vi "Instrument Main Engine.vi"(10 "Parameters":variant, 11 "Process":refnum<class "Process.lvclass">) -> ()   [LabVIEW 2018, in "Instrument Addon Engine.lvlib"]
uses:
  Instrument Addon Engine.lvlib
  Addon Shared/Types/Linked Channel Cluster.ctl
  Addon Shared/Instrument Addon Shared.lvlib
  Addon Shared/Types/Command Parameters.ctl
  <vilib>/NI VeriStand/Custom Device API/Data Reference.ctl
  <vilib>/NI VeriStand/Custom Device API/Custom Device API.lvlib
  Addon Shared/Types/Response Wait Type.ctl
  Addon Shared/Types/Response Parameters.ctl
  Addon Shared/Types/Response RT Configuration Cluster.ctl
  Addon Shared/Types/Message Generation Type.ctl
  Addon Shared/Types/Message Parameters.ctl
  Addon Shared/Types/External Trigger Refs.ctl
  Addon Shared/Types/Compiled Settings.ctl
  niveristand-instrument-addon-custom-device/Source/Addon/Support Libraries/Protections.lvlibp/Parent Protection/Protection.lvclass
  niveristand-instrument-addon-custom-device/Source/Addon/Support Libraries/Protocols.lvlibp/Protocol Parent/Protocol Parent.lvclass
  Types/Commands RT Configuration Cluster.ctl
  <vilib>/NI/NI VeriStand Addon Network Comm/Engine/VeriStand Comm.lvclass
  Addon Shared/Types/Command Channel Index.ctl
  Addon Shared/Types/Command Channel Indeces.ctl
  <vilib>/NI/NIVS Inline Async API/_VS Inline Async API/Process/Process.lvclass
panel:
  in  "error in (no error)":errorcluster
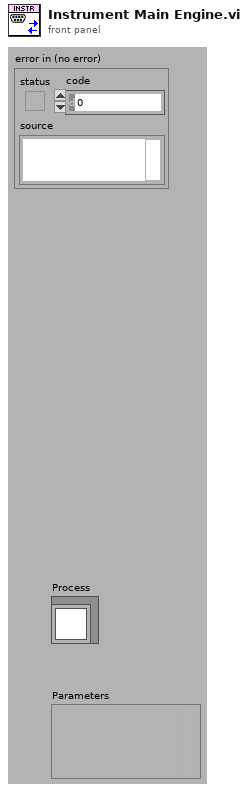
[diagram p1: front panel]
types:
  T1 = typedef "Instrument Addon Engine.lvlib/Commands RT Configuration Cluster.ctl" = cluster{"Compiled":T2, "Protection Settings":refnum<class "Protection.lvclass">[], "Protocol":refnum<class "Protocol Parent.lvclass">}
  T2 = typedef "Instrument Addon Shared.lvlib/Compiled Settings.ctl" = cluster{"Command Parameters":T3[], "Command Indeces":T5[], "MetaData Lookup":variant, "Name":string, "Data Lookup":variant, "Response Parameters":T7[], "Message Generation Settings":T10[], "Wait Value Lookup":variant, "Decimation":u32, "External Channels":T12}
  T3 = typedef "Instrument Addon Shared.lvlib/Command Parameters.ctl" = cluster{"Command":string, "Linked Channels":T4[], "Pad":bool, "Length":u32, "Pad Value":u8}
  T4 = typedef "Instrument Addon Shared.lvlib/Linked Channel Cluster.ctl" = cluster{"Variable Name":string, "GUID":string}
  T5 = typedef "Instrument Addon Shared.lvlib/Command Channel Indeces.ctl" = cluster{"Channels":T6[]}
  T6 = typedef "Instrument Addon Shared.lvlib/Command Channel Index.ctl" = cluster{"Data Index":i32, "Data Length":i32}
  T7 = typedef "Instrument Addon Shared.lvlib/Response RT Configuration Cluster.ctl" = cluster{"Reponse Parameters":T8, "Use?":bool}
  T8 = typedef "Instrument Addon Shared.lvlib/Response Parameters.ctl" = cluster{"Response":string, "Linked Channels":T4[], "Type Value":dbl, "Wait Type":T9, "Use Channel":bool, "Channel Path":string}
  T9 = typedef "Instrument Addon Shared.lvlib/Response Wait Type.ctl" = enum16{"Byte Count", "Wait sec"}
  T10 = typedef "Instrument Addon Shared.lvlib/Message Parameters.ctl" = cluster{"Generation Type":T11, "Period":dbl, "Include Protection":bool, "Type":string}
  T11 = typedef "Instrument Addon Shared.lvlib/Message Generation Type.ctl" = enum16{"Trigger Only", "Periodic & Trigger", "Value Change & Trigger"}
  T12 = typedef "Instrument Addon Shared.lvlib/External Trigger Refs.ctl" = cluster{"Channels":T13[], "Triggers":T13[], "Values":dbl[]}
  T13 = typedef "Custom Device API.lvlib/Data Reference.ctl" = i32
  T14 = typedef "Instrument Addon Engine.lvlib/Engine State Variables.ctl" = cluster{"Comm":refnum<class "VeriStand Comm.lvclass">, "Name":string, "Process":refnum<class "Process.lvclass">, "Statuses":T15, "MetaData":T16, "Triggers":T17, "Periodic Enable":T16, "Data":T15, "Wait":T16, "Wait Values":dbl[], "Data Values":dbl[], "Statuses Values":dbl[], "MetaData Values":dbl[]}
  T15 = typedef "Data Access Engine.lvlib/Data Access Engine.lvclass/Write.DVR.ctl" = refnum<data-value>
  T16 = typedef "Data Access Engine.lvlib/Data Access Engine.lvclass/Read.DVR.ctl" = refnum<data-value>
  T17 = typedef "Data Access Engine.lvlib/Data Access Engine.lvclass/ReadWrite.DVR.ctl" = refnum<data-value>
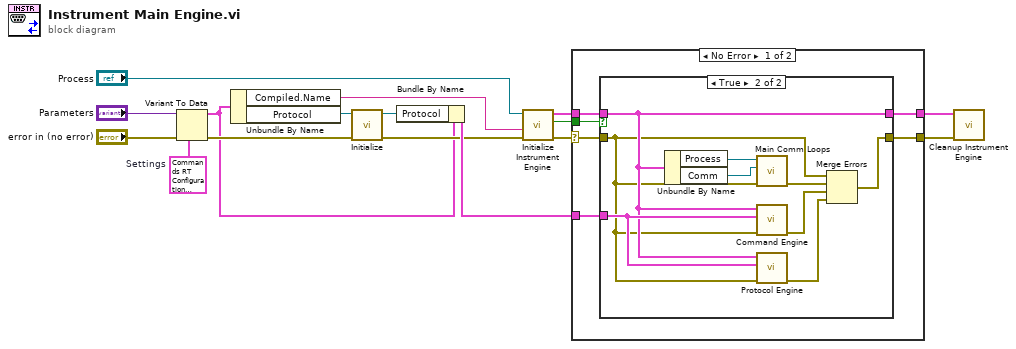
[diagram p0: block diagram]
diagram:
  w4 = T1 {"Compiled"={"Command Parameters"=[], "Command Indeces"=[], "MetaData Lookup"=variant, "Name"="", "Data Lookup"=variant, "Response Parameters"=[], "Message Generation Settings"=[], "Wait Value Lookup"=variant, "Decimation"=0, "External Channels"={"Channels"=[], "Triggers"=[], "Values"=[]}}, "Protection Settings"=[], "Protocol"=refnum}  # Settings
  n1 = Variant To Data(error in="error in (no error)", type=w4, Variant="Parameters") -> (data=w3:T1, error out=w5:errorcluster)
  n2 = Unbundle By Name(w3) -> ("Compiled.Name"=w9:string, "Protocol"=w12:refnum<class "Protocol Parent.lvclass">)
  n3 = call-dynamic "Initialize.vi"("error in (no error)"=w5, "Protocol Parent in"=w12) -> ("error out"=w7:errorcluster, "Protocol Parent out"=w11:refnum<class "Protocol Parent.lvclass">)  [unwired: 8 in]
  n4 = Bundle By Name(cluster=w3, "Protocol"=w11) -> (w10:T1)
  n5 = call "Initialize Instrument Engine.vi"("error in (no error)"=w7, "Name"=w9, "Process"="Process") -> ("error out"=w8:errorcluster, "notification"=w16:bool, "State Variables"=w13:T14)  [unwired: 6 in]
  n6 = case shown="No Error" w8 {
    selector: w8 -> [w20 w35]
    tunnel: w16 -> [w22 _]
    tunnel: [w21 w35] -> w15
    tunnel: w13 -> [w19 w34]
    tunnel: [w18 w34] -> w14
    tunnel: w10 -> [w17 _]
    frame No Error {
      n7 = case shown="True" w22 {
        tunnel: w20 -> [w24 w27]
        tunnel: [w24 w26] -> w21
        tunnel: w19 -> [w23 w32]
        tunnel: [w23 w32] -> w18
        tunnel: w17 -> [_ w33]
        frame False {
        }
        frame True {
          n8 = Unbundle By Name(w32) -> ("Process"=w31:refnum<class "Process.lvclass">, "Comm"=w25:refnum<class "VeriStand Comm.lvclass">)
          n9 = call <vilib>:"Main Comm Loops.vi"("error in (no error)"=w27, "Comm.lvclass"=w25, "Process"=w31) -> ("error out"=w30:errorcluster)  [unwired: 8 in]
          n10 = call "Command Engine.vi"("error in (no error)"=w27, "Settings"=w33, "Global Variables"=w32) -> ("error out"=w29:errorcluster)  [unwired: 8 in]
          n11 = call "Protocol Engine.vi"("error in (no error)"=w27, "Settings"=w33, "State Variables"=w32) -> ("error out"=w28:errorcluster)  [unwired: 8 in]
          n12 = Merge Errors(w27, w30, w29, w28) -> (w26:errorcluster)
        }
      }
    }
    frame Error {
    }
  }
  n13 = call "Cleanup Instrument Engine.vi"("error in (no error)"=w15, "State Variables"=w14) -> ()  [unwired: 10 in]
